vi "Set Temp.vi"(8 "error in (no error)":errorcluster, 10 "Temp C":dbl, 11 "TC-720 in":refnum<class "TC-720.lvclass">) -> (0 "error out":errorcluster, 3 "TC-720 out":refnum<class "TC-720.lvclass">)   [LabVIEW 2023, in "TC-720.lvlib" / "TC-720.lvclass"]
uses:
  TC-720.lvclass
  TC-720.lvclass/TC-720.ctl
  Temperature Controller/Temperature Controller.lvclass
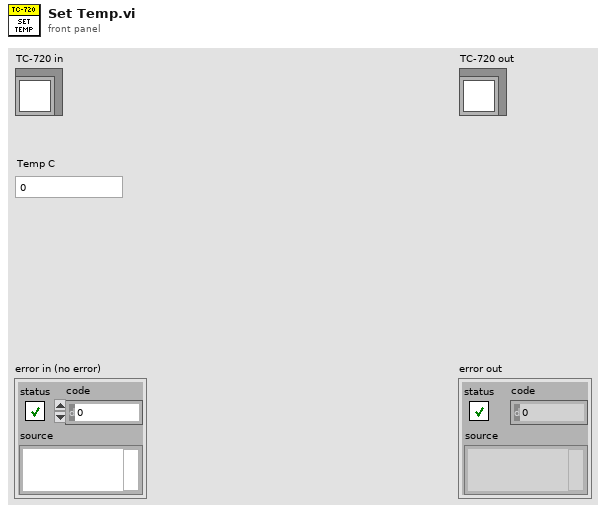
[diagram p1: front panel]
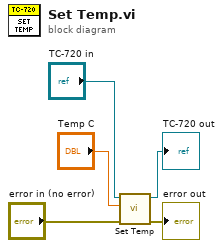
[diagram p0: block diagram]
diagram:
  n1 = call-parent "Set Temp.vi"("error in (no error)"="error in (no error)", "Temp C"="Temp C", "Temperature Controller in"="TC-720 in") -> ("error out"=→"error out":errorcluster, "Temperature Controller out"=→"TC-720 out":refnum<class "TC-720.lvclass">)  [unwired: 7 in]
